vi "mComplete-Event.vi"(8 "Error In":errorcluster) -> (0 "Error Out":errorcluster)   [LabVIEW 2014]
doc: "André Romero - 2023\nandretec@ifsc.usp.br\nIFSC - USP"
uses:
  Global Motors.vi
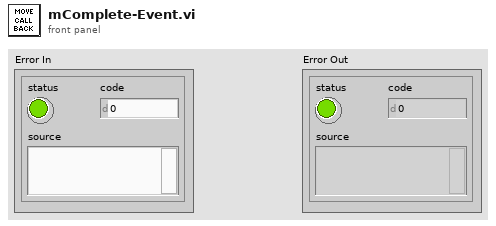
[diagram p1: front panel]
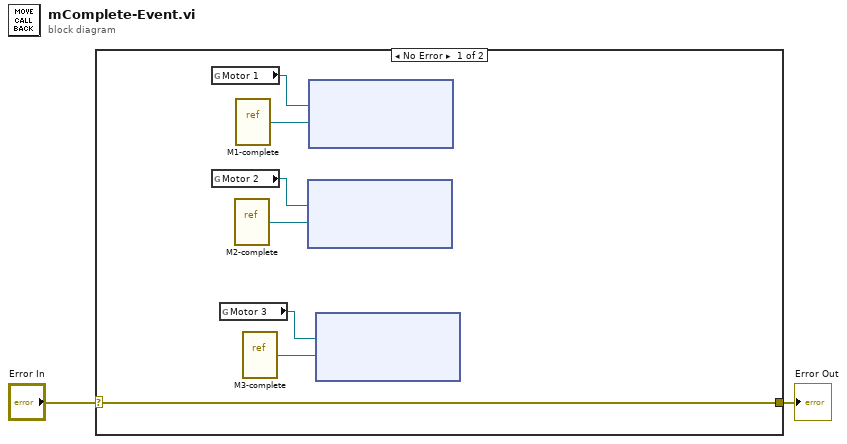
[diagram p0: block diagram]
diagram:
  n1 = case shown="No Error" "Error In" {
    selector: "Error In" -> [w7 w10]
    tunnel: [w7 w10] -> w1
    frame No Error {
      n2 = global read "Global Motors.vi" "Motor 1"() -> (w9:refnum<k7>)
      n3 = global read "Global Motors.vi" "Motor 2"() -> (w8:refnum<k7>)
      n4 = global read "Global Motors.vi" "Motor 3"() -> (w6:refnum<k7>)
      n5 = vi-ref "M2-complete.vi"() -> ("vi reference"=w4:refnum<vi>)
      n6 = vi-ref "M1-complete.vi"() -> ("vi reference"=w5:refnum<vi>)
      n7 = vi-ref "M3-complete.vi"() -> ("vi reference"=w3:refnum<vi>)
      n8 = node(w8, w4) -> ()  [unwired: 3 in, 2 out]
      n9 = node(w9, w5) -> ()  [unwired: 3 in, 2 out]
      n10 = node(w6, w3) -> ()  [unwired: 3 in, 2 out]
    }
    frame Error {
    }
  }
  "Error Out" <- w1
